vi "host.vi"() -> ()   [LabVIEW 2020]
uses:
  <vilib>/FPGAPlugInAG/cRIO-9035/niLvFpga_Open_cRIO-9035.vi
  <vilib>/rvi/interface/common/dynamic/niFpgaDynamicAddResources.vi
  <vilib>/Utility/error.llb/Error Cluster From Error Code.vi
  <vilib>/rvi/errors/niLvFpgaAdjustHostInterfaceError.vi
  <vilib>/FPGAPlugInAG/Dynamic/niLvFpga_Run_Dynamic.vi
  <vilib>/FPGAPlugInAG/Dynamic/niLvFpga_Close_Dynamic.vi
  <vilib>/rvi/interface/nirviOpenFPGA/nirviOpenFPGA.xnode
  FPGA Bitfiles/firstfpgaapplica_FPGATarget_FFT_Un-ypgSOa9s.lvbitx
  FFT.vi
  <vilib>/rvi/interface/nirviMethod/nirviMethod.xnode
  <vilib>/rvi/interface/nirviCloseFPGA/nirviCloseFPGA.xnode
  <vilib>/rvi/errors/niLvFpgaMergeErrorWithErrorCode.vi
  <vilib>/FPGAPlugInAG/Dynamic/niLvFpga_ReadFifo_Dynamic.vi
  <vilib>/FPGAPlugInAG/Dynamic/niLvFpga_WriteFifo_Dynamic.vi
panel:
  out "end tick":fxp<+/-,32,16>[](array[numeric])
  out "start ticka":fxp<+/-,32,16>[](array[numeric])
  out "Waveform Graph":dbl[][](graph)
  out "XY Graph":T1(graph)
  out "Array":fxp<+/-,32,16>[](array[numeric])
  out "MLP 1 size(s)":i32
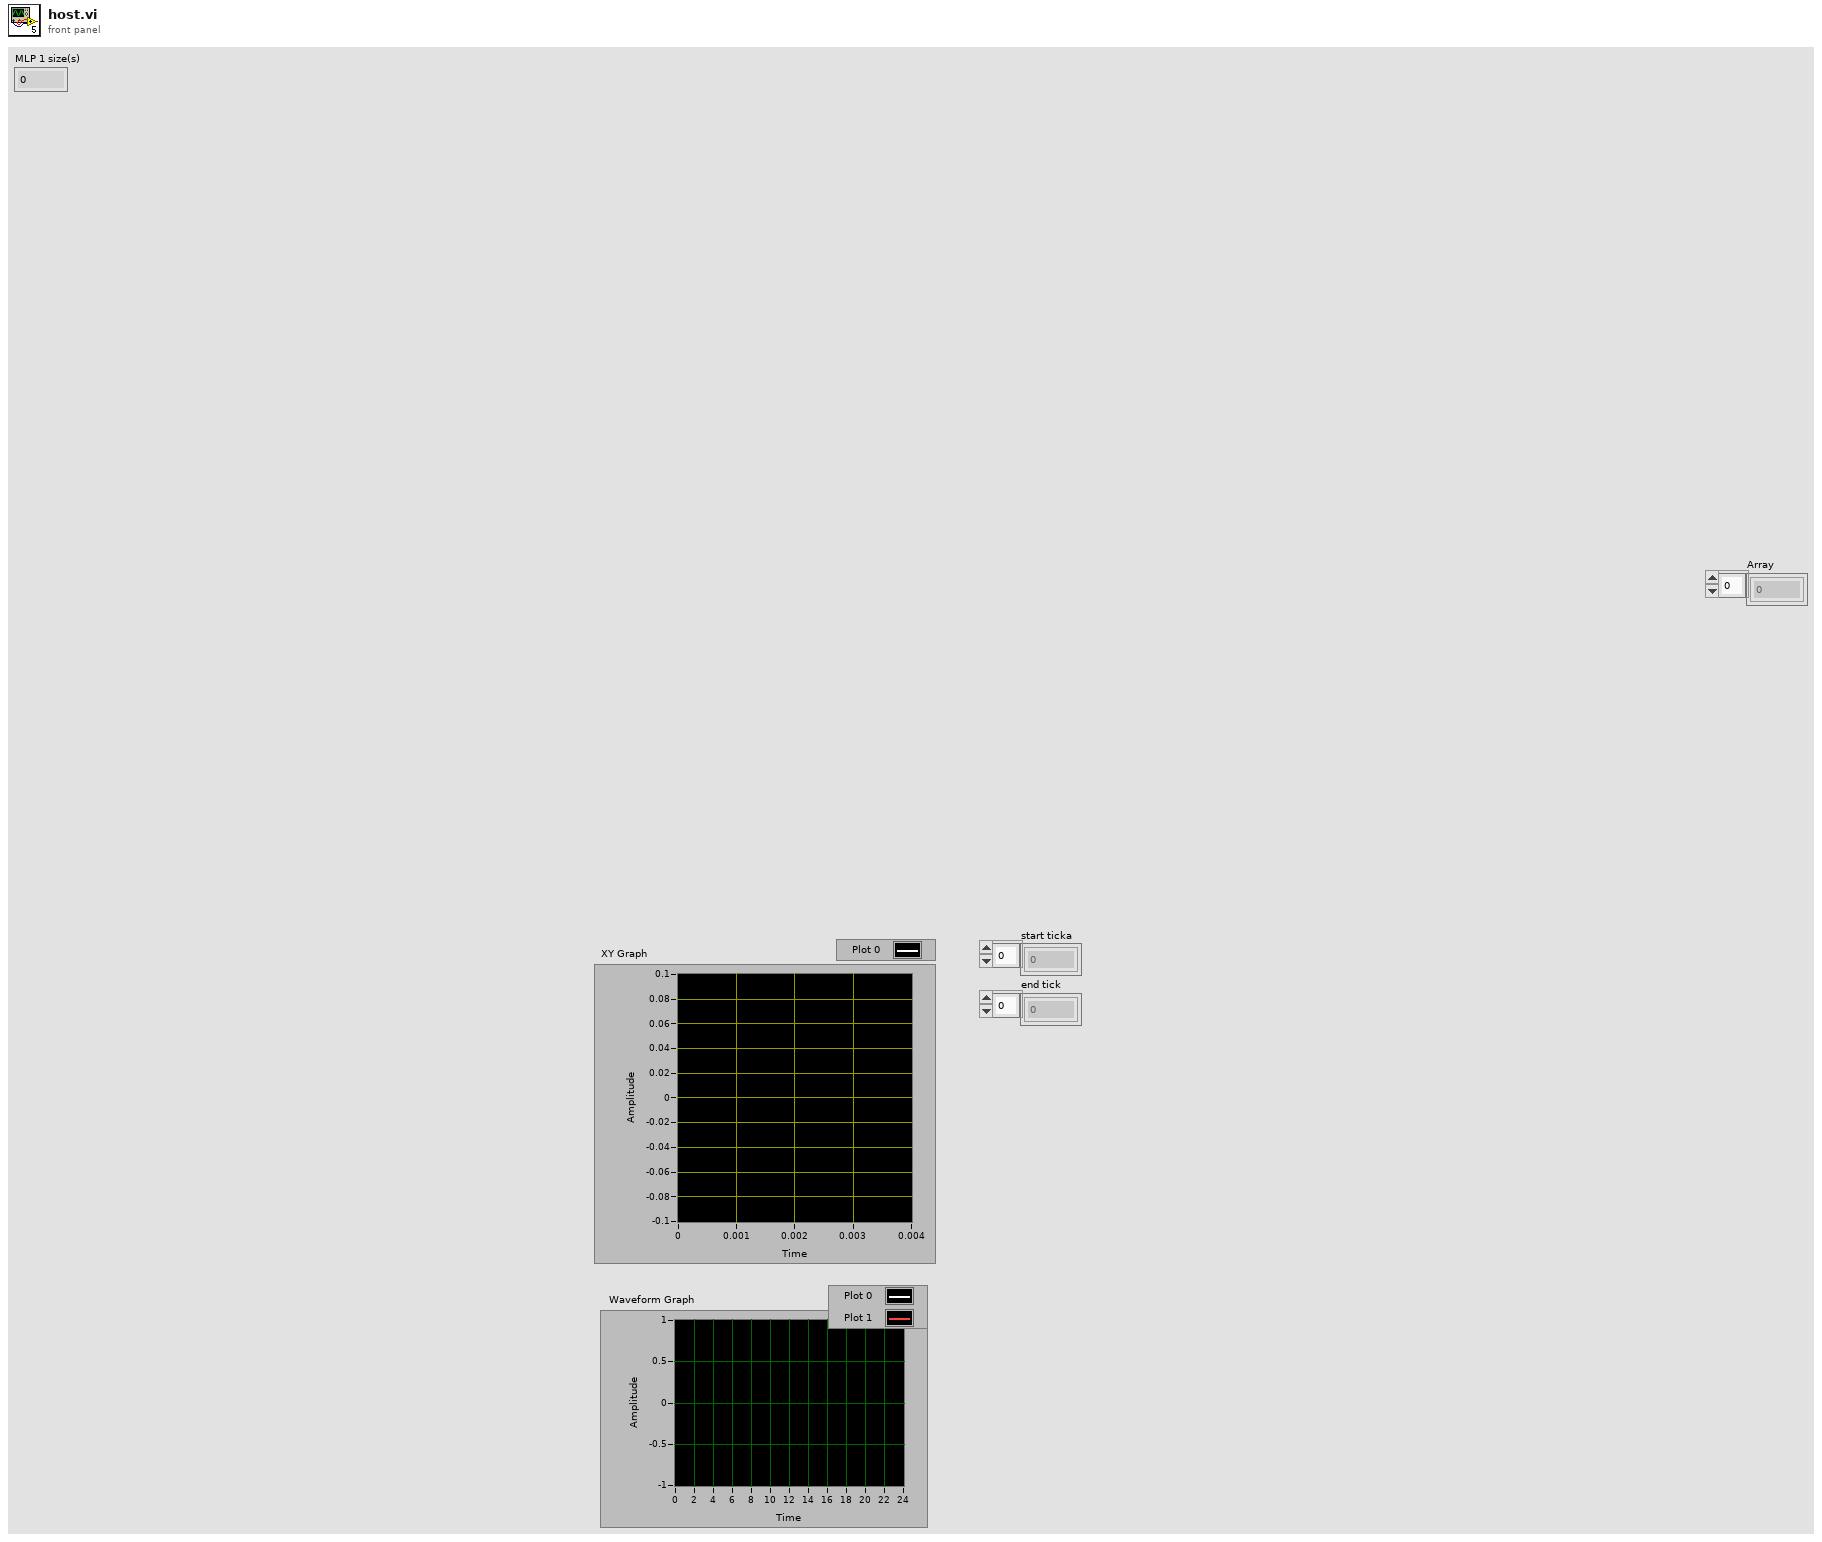
[diagram p1: front panel]
types:
  T1 = cluster{"array type (2D Dbl)":dbl[], "array type (2D Dbl)":dbl[]}
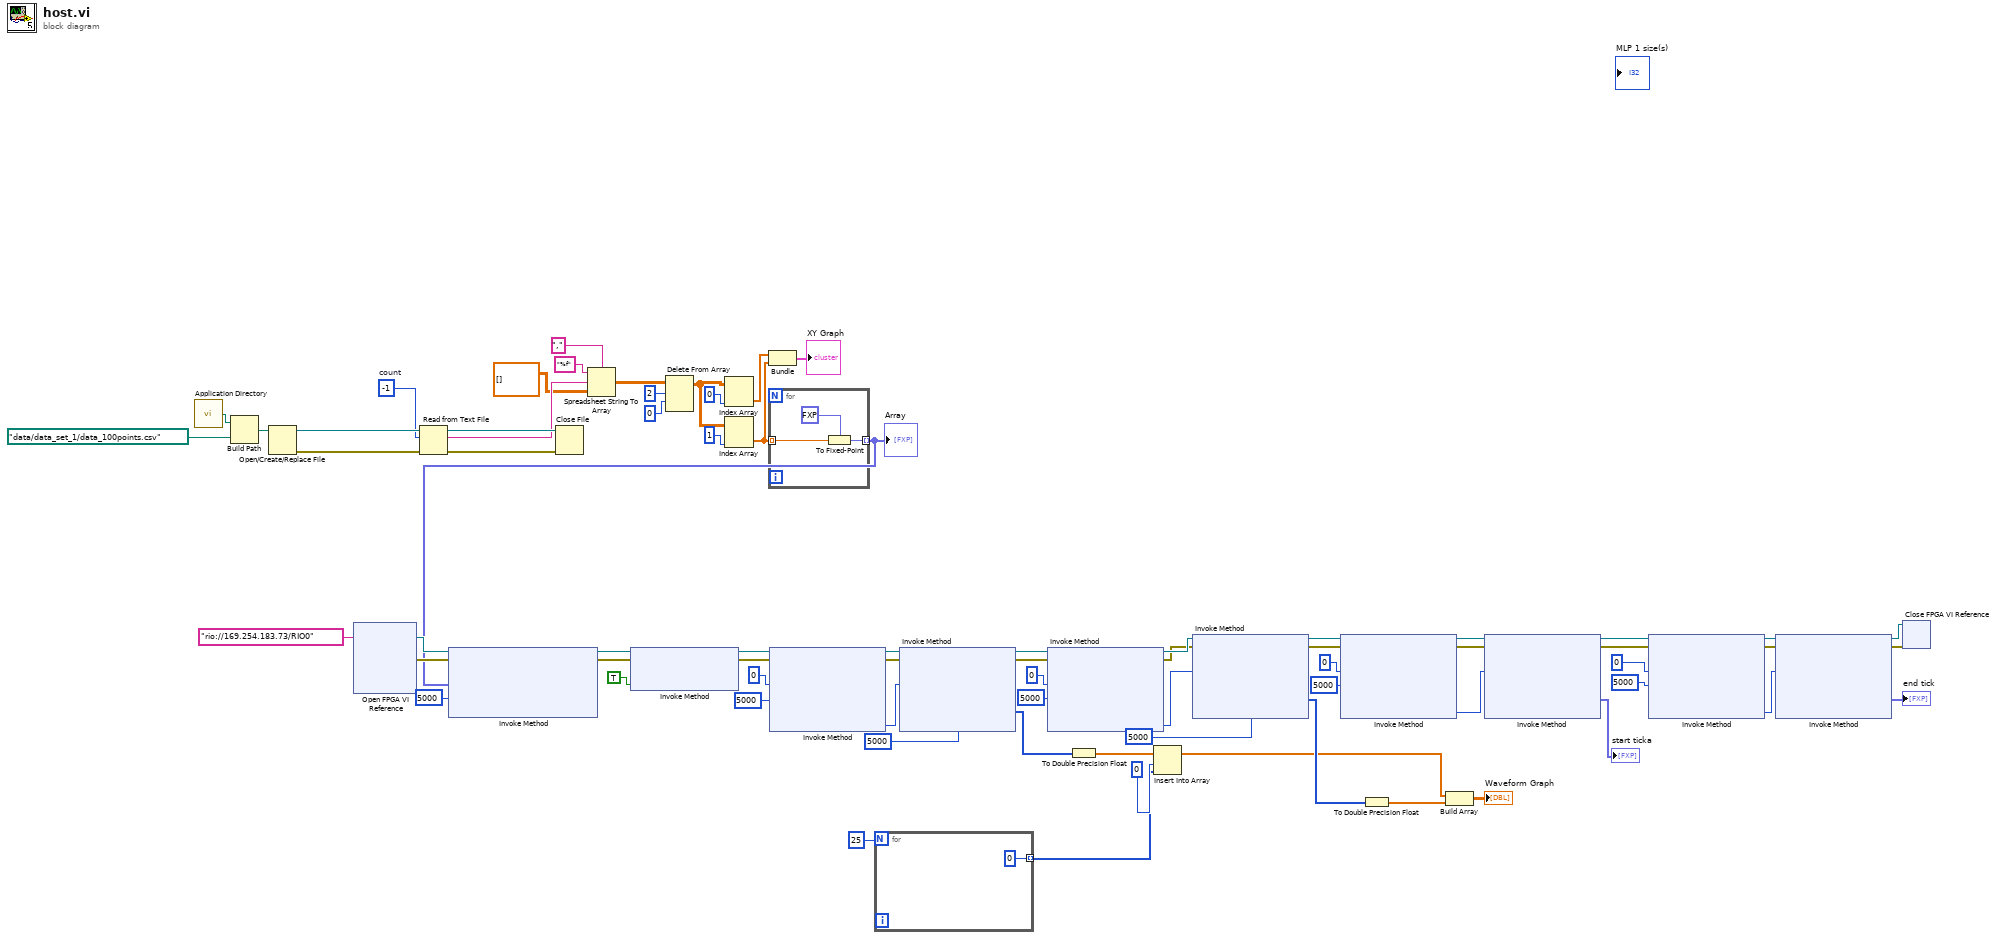
[diagram p0: block diagram]
diagram:
  w63 = -1  # count
  n1 = call <vilib>:"Application Directory.vi"() -> ("Application Directory"=w67:path)
  n2 = Build Path(base path=w67, name or relative path=path "data/data_set_1/data_100points.csv" ("default name")) -> (appended path=w66:path)
  n3 = Open/Create/Replace File(file path (use dialog)=w66) -> (refnum out=w71:refnum<file>, error out=w72:errorcluster)  [unwired: 5 in, 1 out]
  n4 = xnode "Open FPGA VI Reference"("resource name"=tag "rio://169.254.183.73/RIO0") -> ("FPGA VI Reference Out"=w51:refnum<k20>, "error out"=w50:errorcluster)  [unwired: 1 in]
  n5 = Read from Text File(file (use dialog)=w71, count=w63, error in=w72) -> (refnum out=w70:refnum<file>, text=w68:string, error out=w69:errorcluster)  [unwired: 1 in, 1 out]
  n6 = Close File(refnum=w70, error in=w69) -> ()  [unwired: 2 out]
  n7 = Spreadsheet String To Array(delimiter (Tab)=",", format string="%f", spreadsheet string=w68, array type (2D Dbl)=dbl[][] []) -> (array=w60:dbl[][])
  n8 = Delete From Array(array=w60, length=2, index (row)=0) -> (array with subset deleted=w54:dbl[][])  [unwired: 1 in, 1 out]
  n9 = Index Array(array=w54, index (col)=0 ("disabled index (col)")) -> (element=w52:dbl[])  [unwired: 1 in]
  n10 = Index Array(array=w54, index (col)=1 ("disabled index (col)")) -> (element=w56:dbl[])  [unwired: 1 in]
  n11 = Bundle("array type (2D Dbl)"=w52, "array type (2D Dbl)"=w56) -> (→"XY Graph":T1)  [unwired: 1 in]
  n12 = for {
    tunnel: [w74] -> w49 mode=indexing
    tunnel: w56 -> [w73] mode=indexing
    n13 = To Fixed-Point(fixed-point type=fxp<+/-,32,16> 0.0 ("f"), number=w73) -> (fixed-point=w74:fxp<+/-,32,16>)
  }
  "Array" <- w49
  n14 = xnode "Invoke Method"("FPGA VI Reference In"=w51, "error in"=w50, "Data"=w49, "Timeout (ms)"=5000) -> ("FPGA VI Reference Out"=w47:refnum<k20>, "error out"=w46:errorcluster)  [unwired: 1 out]
  n15 = xnode "Invoke Method"("FPGA VI Reference In"=w47, "error in"=w46, "Wait Until Done (F)"=TRUE) -> ("FPGA VI Reference Out"=w45:refnum<k20>, "error out"=w44:errorcluster)
  n16 = xnode "Invoke Method"("FPGA VI Reference In"=w45, "error in"=w44, "Number of Elements"=u32 0, "Timeout (ms)"=5000) -> ("FPGA VI Reference Out"=w43:refnum<k20>, "error out"=w42:errorcluster, "Elements Remaining"=w36:u32)  [unwired: 1 out]
  n17 = for {
    N: 25 -> [_]
    tunnel: [0] -> w26 mode=indexing
  }
  n18 = xnode "Invoke Method"("FPGA VI Reference In"=w43, "error in"=w42, "Number of Elements"=w36, "Timeout (ms)"=5000) -> ("FPGA VI Reference Out"=w39:refnum<k20>, "error out"=w38:errorcluster, "Data"=w32:i32[])  [unwired: 1 out]
  n19 = xnode "Invoke Method"("FPGA VI Reference In"=w39, "error in"=w38, "Number of Elements"=u32 0, "Timeout (ms)"=5000) -> ("FPGA VI Reference Out"=w41:refnum<k20>, "error out"=w40:errorcluster, "Elements Remaining"=w34:u32)  [unwired: 1 out]
  n20 = To Double Precision Float(number=w32) -> (double precision float=w30:dbl[])
  n21 = Insert Into Array(array=w30, index=0, new element=w26) -> (w28:dbl[])
  n22 = xnode "Invoke Method"("FPGA VI Reference In"=w41, "error in"=w40, "Number of Elements"=w34, "Timeout (ms)"=5000) -> ("FPGA VI Reference Out"=w23:refnum<k20>, "error out"=w22:errorcluster, "Data"=w31:i32[])  [unwired: 1 out]
  n23 = xnode "Invoke Method"("FPGA VI Reference In"=w23, "error in"=w22, "Number of Elements"=u32 0, "Timeout (ms)"=5000) -> ("FPGA VI Reference Out"=w21:refnum<k20>, "error out"=w20:errorcluster, "Elements Remaining"=w13:u32)  [unwired: 1 out]
  n24 = To Double Precision Float(number=w31) -> (double precision float=w27:dbl[])
  n25 = Build Array(w28, w27) -> (→"Waveform Graph":dbl[][])
  n26 = xnode "Invoke Method"("FPGA VI Reference In"=w21, "error in"=w20, "Number of Elements"=w13) -> ("FPGA VI Reference Out"=w19:refnum<k20>, "error out"=w18:errorcluster, "Data"=→"start ticka":fxp<+/-,32,16>[])  [unwired: 1 in, 1 out]
  n27 = xnode "Invoke Method"("FPGA VI Reference In"=w19, "error in"=w18, "Number of Elements"=u32 0, "Timeout (ms)"=5000) -> ("FPGA VI Reference Out"=w17:refnum<k20>, "error out"=w16:errorcluster, "Elements Remaining"=w11:u32)  [unwired: 1 out]
  n28 = xnode "Invoke Method"("FPGA VI Reference In"=w17, "error in"=w16, "Number of Elements"=w11) -> ("FPGA VI Reference Out"=w15:refnum<k20>, "error out"=w14:errorcluster, "Data"=→"end tick":fxp<+/-,32,16>[])  [unwired: 1 in, 1 out]
  n29 = xnode "Close FPGA VI Reference"("FPGA VI Reference In"=w15, "error in"=w14) -> ()  [unwired: 1 out]
